vi "Get Absolute Source Dir Path.vi"() -> (3 "source dir":path)   [LabVIEW 2020]
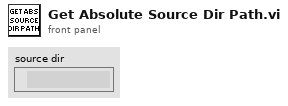
[diagram p1: front panel]
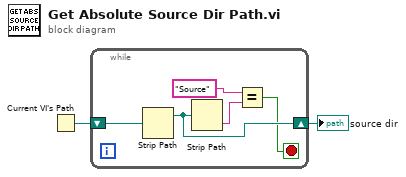
[diagram p0: block diagram]
diagram:
  n1 = Current VI's Path() -> (path=w2:path)
  n2 = while {
    shift-right: [w6] -> w1
    shift-left: w2 -> [w7]
    stop <- w3 stop-if-true
    # "Find the source dir"
    n3 = Strip Path(path=w7) -> (stripped path=w6:path)  [unwired: 1 out]
    n4 = Strip Path(path=w6) -> (name=w5:string)  [unwired: 1 out]
    n5 = Equal?(x="Source", y=w5) -> (x = y?=w3:bool)
  }
  "source dir" <- w1
